vi "Run Step.vi"(7 "New Step":bool, 8 "error in (no error)":errorcluster, 9 "result allocation":T1, 10 "parameters":T1, 11 "Update Tag in":refnum<class "Update Tag.lvclass">) -> (0 "error out":errorcluster, 1 "results":T1, 2 "parameter allocation":T1, 3 "Update Tag out":refnum<class "Update Tag.lvclass">, 4 "Completed":bool)   [LabVIEW 2015, in "Update Tag.lvclass"]
uses:
  Update Tag.lvclass
  <vilib>/NI/Tag Bus/table/data table.ctl
  Update Tag.lvclass/Update Tag.ctl
  <vilib>/NI/Tag Bus/table/data polymorphs/write one/write Double.vi
  <vilib>/NI/Tag Bus/table/data polymorphs/write one/write Boolean.vi
  <vilib>/NI/Tag Bus/table/data table.lvlib
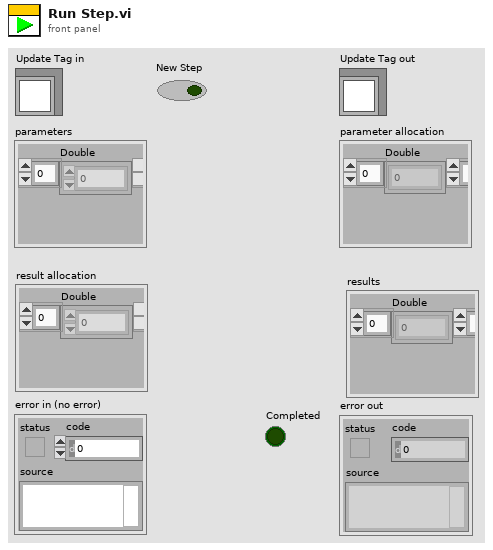
[diagram p1: front panel]
types:
  T1 = typedef "tag bus.lvlib/data table.lvlib/data table.ctl" = cluster{"Double":dbl[], "Single":sgl[], "I64":i64[], "I32":i32[], "I16":i16[], "I8":i8[], "U64":u64[], "U32":u32[], "U16":u16[], "U8":u8[], "Boolean":bool[], "String":string[], "Array of Double":cluster{"DBL Array":dbl[]}[], "Array of Single":cluster{"SGL Array":sgl[]}[], "Array of I64":cluster{"I64 Array":i64[]}[], "Array of I32":cluster{"I32 Array":i32[]}[], "Array of I16":cluster{"I16 Array":i16[]}[], "Array of I8":cluster{"I8 Array":i8[]}[], "Array of U64":cluster{"U64 Array":u64[]}[], "Array of U32":cluster{"U32 Array":u32[]}[], "Array of U16":cluster{"U16 Array":u16[]}[], "Array of U8":cluster{"U8 Array":u8[]}[], "Array of Boolean":cluster{"Boolean Array":bool[]}[], "Array of String":cluster{"String Array":string[]}[]}
  T2 = typedef "tag bus.lvlib/tag descriptor.lvclass/Data Type.ctl" = enum16{"Double", "Single", "I64", "I32", "I16", "I8", "U64", "U32", "U16", "U8", "Boolean", "String", "Array of Double", "Array of Single", "Array of I64", "Array of I32", "Array of I16", "Array of I8", "Array of U64", "Array of U32", "Array of U16", "Array of U8", "Array of Boolean", "Array of String"}
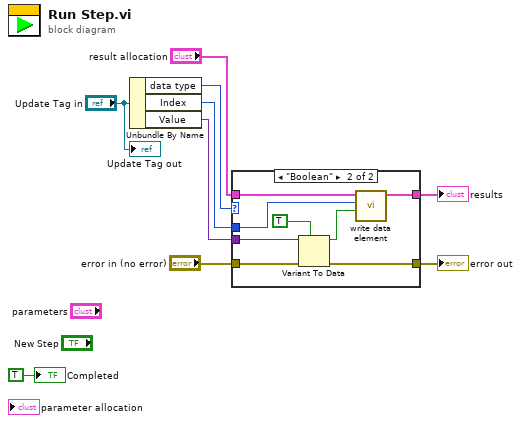
[diagram p0: block diagram]
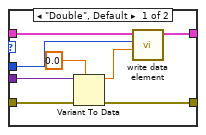
[diagram p2: hidden frame]
diagram:
  n1 = Unbundle By Name("Update Tag in") -> ("data type"=w7:T2, "Index"=w6:i32, "Value"=w4:variant)
  n2 = case shown="\"Boolean\"" w7 {
    tunnel: w6 -> [w16 w24]
    tunnel: "result allocation" -> [w17 w25]
    tunnel: w4 -> [w15 w23]
    tunnel: [w12 w21] -> w3
    tunnel: "error in (no error)" -> [w11 w20]
    tunnel: [w10 w19] -> w1
    frame "Double", Default {
      n3 = Variant To Data(error in=w11, type=0.0 ("value"), Variant=w15) -> (data=w13:dbl, error out=w10:errorcluster)
      n4 = call-poly <vilib>:"write data element.vi"("value"=w13, "index"=w16, "data table in"=w17) -> ("data table out"=w12:T1)  [unwired: 8 in]
    }
    frame "Boolean" {
      n5 = Variant To Data(error in=w20, type=TRUE ("Completed"), Variant=w23) -> (data=w22:bool, error out=w19:errorcluster)
      n6 = call-poly <vilib>:"write data element.vi"("value"=w22, "index"=w24, "data table in"=w25) -> ("data table out"=w21:T1)  [unwired: 8 in]
    }
  }
  "error out" <- w1
  "results" <- w3
  "Update Tag out" <- "Update Tag in"
  "Completed" <- TRUE ("Completed")
